vi "Test Process Error Flow Through.vi"(8 "error in (no error)":errorcluster, 11 "Process Test in":refnum<class "Process Test.lvclass">) -> (0 "error out":errorcluster, 3 "Process Test out":refnum<class "Process Test.lvclass">)   [LabVIEW 2020, in "Process Test.lvclass"]
uses:
  Process Test.lvclass
  C:/Program Files (x86)/National Instruments/LabVIEW 2020/vi.lib/Asteme/LUnit/Test Case.lvclass
  Framework/Process/Process.lvclass/Process.ctl
  <vilib>/Asteme/LUnit/Test Case.lvclass/Test Case.ctl
  <vilib>/Asteme/LUnit/LUnit Assertion Result.lvclass/LUnit Assertion Result.ctl
  Framework/Process/Public/Lifecycle/Get Lifecycle State.vi
  Framework/Process/Private/SubVIs/Wait for finish.vi
  Framework/Process/Protected/Messaging/Enqueue Message.vi
  Framework/Process/Private/SubVIs/Set Lifecycle State.vi
  <vilib>/Asteme/LUnit/Palette/Pass If.vi
  <vilib>/Asteme/LUnit/Set Assertion Type.vi
  <vilib>/Asteme/LUnit/Palette/Pass.vi
  <vilib>/Asteme/LUnit/Palette/Fail.vi
  <vilib>/Asteme/LUnit/Variant to string.vi
  <vilib>/Utility/error.llb/Clear Errors.vi
  <vilib>/Asteme/LUnit/LUnit Write Assertion Type.vi
  <vilib>/Asteme/LUnit/Add test result.vi
  <vilib>/Asteme/LUnit/LUnit Write Passed.vi
  <vilib>/Asteme/LUnit/LUnit Get Test Case.vi
  <vilib>/Asteme/LUnit/Assertion Result/LUnit Get Test Name.vi
  <vilib>/Asteme/LUnit/LUnit Write Message.vi
  <vilib>/Asteme/LUnit/LUnit Write Description.vi
  <vilib>/Asteme/LUnit/Read Test Case Name.vi
  <vilib>/Utility/error.llb/Error Cluster From Error Code.vi
  <vilib>/Utility/Data Type/Get Type Information.vi
  <vilib>/Utility/LVClass/Get LV Class Name.vi
  <vilib>/ErrorRing/Error Ring.xnode
  <vilib>/Asteme/LUnit/LUnit Assertion Result.lvclass
  Framework/Process/Process.lvclass
  <vilib>/Asteme/LUnit/Test Case.lvclass
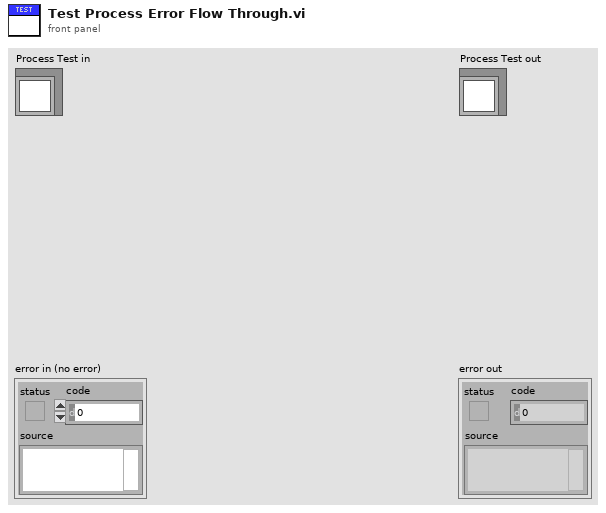
[diagram p1: front panel]
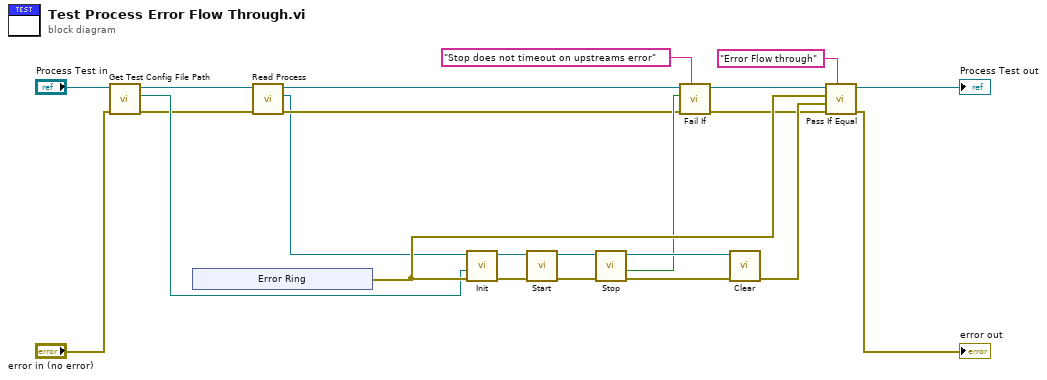
[diagram p0: block diagram]
diagram:
  n1 = call-dynamic "Get Test Config File Path.vi"("error in (no error)"="error in (no error)", "Base Class Test in"="Process Test in") -> ("error out"=w5:errorcluster, "Test config path"=w11:path, "Base Class Test out"=w3:refnum<class "Process Test.lvclass">)  [unwired: 7 in]
  n2 = xnode "Error Ring"() -> ("error out"=w13:errorcluster)
  n3 = call "Read Process.vi"("error in (no error)"=w5, "Process Test in"=w3) -> ("error out"=w4:errorcluster, "Process.lvclass"=w1:refnum<class "Process.lvclass">, "Process Test out"=w2:refnum<class "Process Test.lvclass">)  [unwired: 7 in]
  n4 = call-dynamic "Init.vi"("error in (no error)"=w13, "Config File Path"=w11, "Process In"=w1) -> ("error out"=w12:errorcluster, "Process Out"=w16:refnum<class "Process.lvclass">)  [unwired: 7 in]
  n5 = call "Start.vi"("error in (no error)"=w12, "Process In"=w16) -> ("error out"=w22:errorcluster, "Process Out"=w23:refnum<class "Process.lvclass">)  [unwired: 8 in]
  n6 = call "Stop.vi"("error in (no error)"=w22, "Process In"=w23) -> ("error out"=w18:errorcluster, "timed out?"=w7:bool, "Process Out"=w14:refnum<class "Process.lvclass">)  [unwired: 7 in]
  n7 = call <vilib>:"Fail If.vi"("Description"="Stop does not timeout on upstreams error", "error in (no error)"=w4, "Fail?"=w7, "Test Case In"=w2) -> ("error out"=w8:errorcluster, "Test Case Out"=w9:refnum<class "Process Test.lvclass">)  [unwired: 6 in]
  n8 = call-dynamic "Clear.vi"("error in (no error)"=w18, "Process In"=w14) -> ("error out"=w15:errorcluster)  [unwired: 8 in, 1 out]
  n9 = call <vilib>:"Pass If Equal.vi"("Description"="Error Flow through", "error in (no error)"=w8, "Actual"=w15, "Expected"=w13, "Test Case In"=w9) -> ("error out"=→"error out":errorcluster, "Test Case Out"=→"Process Test out":refnum<class "Process Test.lvclass">)  [unwired: 5 in]
